vi "MirrorPositions.vi"(6 "all status array":refnum<vi>, 8 "Array":T1(array[cluster]), 9 "reference":refnum<vi>, 10 "Multicolumn Listbox 2":refnum<vi>, 11 "Array in":refnum<vi>) -> ()   [LabVIEW 2013]
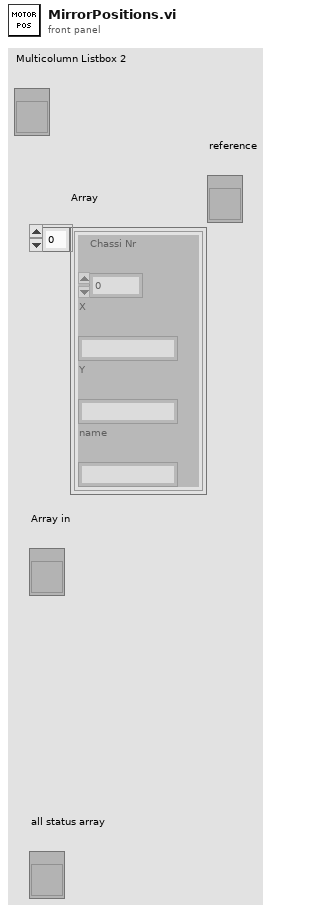
[diagram p1: front panel]
types:
  T1 = cluster{"Chassi Nr":i32, "X":string, "Y":string, "name":string}[]
  T2 = enum32{"Main", "Status", "Position", "Position 2", "Temp", "Network", "Internal", "MotorSettings"}
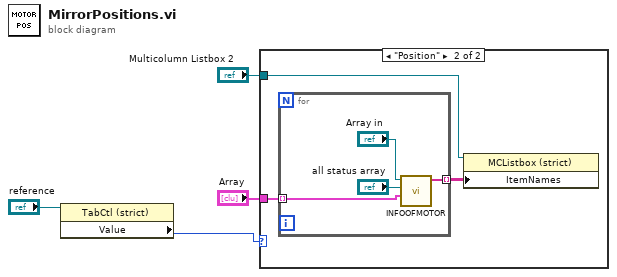
[diagram p0: block diagram]
diagram:
  n1 = property class="TabCtl (strict)"(reference="reference") -> ("Value"=w2:T2)  [unwired: 1 in, 2 out]
  n2 = case shown="\"Position\"" w2 {
    tunnel: "Array" -> [_ w7]
    tunnel: "Multicolumn Listbox 2" -> [_ w6]
    frame "Main", Default {
    }
    frame "Position" {
      n3 = for {
        tunnel: w7 -> [w11] mode=indexing
        tunnel: [w8] -> w5 mode=indexing
        n4 = call "INFOOFMOTOR.vi"("input cluster"=w11, "reference in"="all status array", "Array in"="Array in") -> ("Mirror Info"=w8:string[])  [unwired: 8 in]
      }
      n5 = property class="MCListbox (strict)"(reference=w6, "ItemNames"=w5) -> ()  [unwired: 1 in, 2 out]
    }
  }
